vi "Add_Post_Install_Step.vi"(8 "error in (no error)":errorcluster, 11 "IB_Source_File_Web_Service in":refnum<class "IB_Source_File_Web_Service.lvclass">) -> (0 "error out":errorcluster, 1 "add?":bool, 2 "Pre_Uninstall_Step":refnum<class "IB_Post_Install_Step.lvclass">, 3 "Post_Install_Step":refnum<class "IB_Post_Install_Step.lvclass">)   [LabVIEW 2020, in "IB_Source_File_Web_Service.lvclass"]
uses:
  <vilib>/AppBuilder/IB_Classes/Source/File_Web_Service/IB_Source_File_Web_Service.lvclass
  <vilib>/AppBuilder/IB_Classes/Source/File_Web_Service/IB_Source_File_Web_Service.lvclass/IB_Source_File_Web_Service.ctl
  <vilib>/AppBuilder/IB_Classes/Source/IB_Source.lvclass
  e:/builds/penguin/labview/branches/2020/dev/dist/vi.lib/AppBuilder/IB_Classes/Source/File/IB_Source_File.lvclass
  e:/builds/penguin/labview/branches/2020/dev/dist/vi.lib/AppBuilder/IB_Classes/Source/IB_Source.lvclass
  e:/builds/penguin/labview/branches/2020/dev/dist/vi.lib/AppBuilder/IB_Classes/Source/File_Web_Service/IB_Source_File_Web_Service.lvclass
  <vilib>/AppBuilder/IB_Classes/Post_Install_Step/IB_Post_Install_Step.lvclass
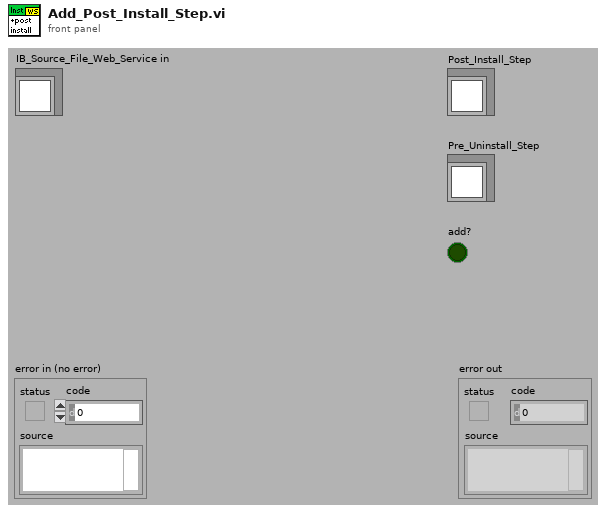
[diagram p1: front panel]
types:
  T1 = typedef "IB_Source.ctl" = cluster{"name":string, "sourceTag":string, "destTag":string, "path":path, "eng_installPath":string, "UI_inBuild?":bool, "str ref?":bool}
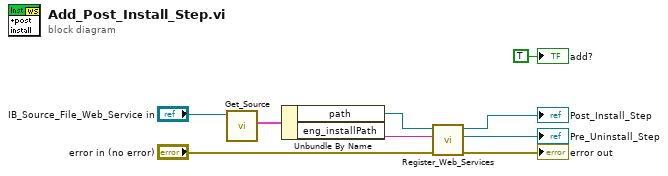
[diagram p0: block diagram]
diagram:
  n1 = call <vilib>:"Get_Source.vi"("IB_Source in"="IB_Source_File_Web_Service in") -> ("data"=w8:T1)  [unwired: 8 in, 2 out]
  n2 = Unbundle By Name(w8) -> ("path"=w6:path, "eng_installPath"=w7:string)
  n3 = call <vilib>:"Register_Web_Services.vi"("error in"="error in (no error)", "eng_installPath"=w7, "source path"=w6) -> ("error out"=→"error out":errorcluster, "Pre_Uninstall_Step"=→"Pre_Uninstall_Step":refnum<class "IB_Post_Install_Step.lvclass">, "Post_Install_Step"=→"Post_Install_Step":refnum<class "IB_Post_Install_Step.lvclass">)  [unwired: 6 in]
  "add?" <- TRUE ("add?")
